vi "NewOrObtainQueue__slk__QSM-PC (String).vi"(8 "error in (no error)":errorcluster, 11 "queue name in":string) -> (0 "error out":errorcluster, 3 "queue out":refnum<queue>)   [LabVIEW 2016, in "QSM-PC (String).lvlib"]
doc: "Creates a queue if the queue is not exist, or returen queue refnum if the queue is exist."
uses:
  Library/QSM-PC (String).lvlib
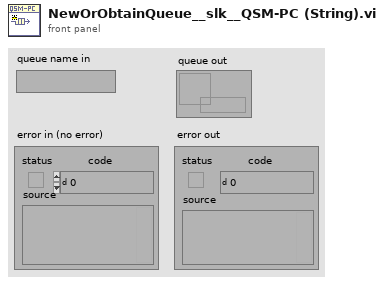
[diagram p1: front panel]
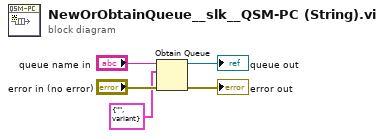
[diagram p0: block diagram]
diagram:
  n1 = Obtain Queue(name (unnamed)="queue name in", element data type=cluster{"State":string, "Data":variant} {"State"="", "Data"=variant} ("Element"), error in (no error)="error in (no error)") -> (queue out=→"queue out":refnum<queue>, error out=→"error out":errorcluster)  [unwired: 2 in, 1 out]
